vi "Cleanup Session.vi"(8 "error in":errorcluster, 11 "Plugin in":refnum<class "Waterfall.lvclass">) -> (0 "error out":errorcluster, 3 "Plugin out":refnum<class "Waterfall.lvclass">)   [LabVIEW 2024, in "Waterfall.lvlib" / "Waterfall.lvclass"]
uses:
  Waterfall.lvclass
  Waterfall.lvclass/Waterfall.ctl
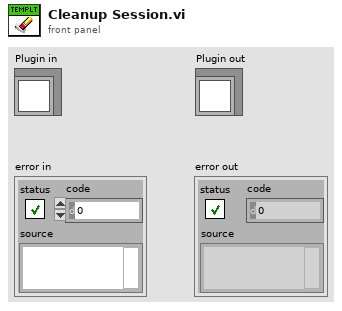
[diagram p1: front panel]
types:
  T1 = enum32{"Invalid", "Standard", "Closed", "Hidden", "Minimized", "Maximized"}
  T2 = typedef "Waterfall.lvlib/Waterfall.lvclass/Waterfall Data.ctl" = cluster{"First Time":bool, "Show Waterfall Button Clicked":bool, "Data to Process":dbl, "Slice":dbl, "window":T3, "averaging parameters":cluster{"averaging mode":enum16{"No averaging", "Vector averaging", "RMS averaging", "Peak hold"}, "weighting mode":enum16{"Linear", "Exponential"}, "number of averages":u32}, "Waterfall VI Ref":refnum<vi>, "Signal":waveform(dbl)}
  T3 = typedef "NI_AALPro.lvlib/windowTd.ctl" = u32
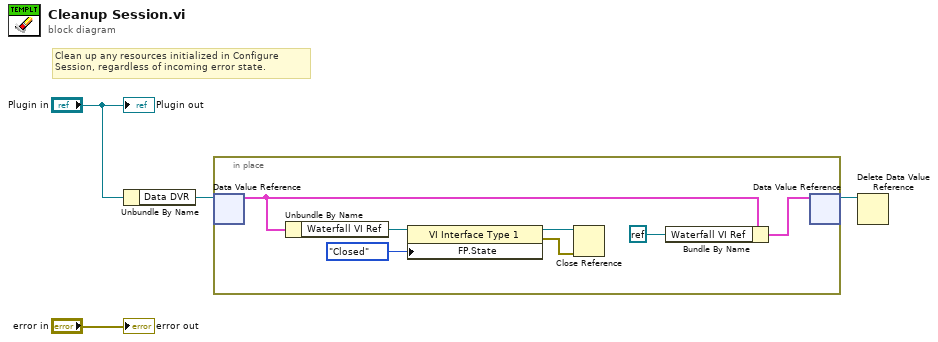
[diagram p0: block diagram]
diagram:
  # "Clean up any resources initialized in Configure Session, regardless of incoming error state."
  n1 = Unbundle By Name("Plugin in") -> ("Data DVR"=w3:refnum<data-value>)
  n2 = in-place {
    n3 = in-place-dvr #1(w3) -> (w11:T2)  [unwired: 1 out]
    n4 = Unbundle By Name(w11) -> ("Waterfall VI Ref"=w8:refnum<vi>)
    n5 = property class="VI Interface Type 1"(reference=w8, "FP.State"=T1."Closed" ("Front Panel Window:State")) -> (reference out=w7:refnum<vi>, error out=w5:errorcluster)  [unwired: 1 in]
    n6 = Close Reference(reference=w7, error in (no error)=w5) -> ()  [unwired: 1 out]
    n7 = Bundle By Name(cluster=w11, "Waterfall VI Ref"=refnum<k0> refnum) -> (w9:T2)
    n8 = in-place-dvr #1(w9) -> (w2:refnum<data-value>)  [unwired: 1 out]
  }
  n9 = Delete Data Value Reference(data value reference=w2) -> ()  [unwired: 1 in, 2 out]
  "error out" <- "error in"
  "Plugin out" <- "Plugin in"
